vi "Close Notifiers.vi"(8 "error in":errorcluster, 11 "Notifiers":T1) -> (0 "error out":errorcluster)   [LabVIEW 2015, in "Notifiers.lvlib"]
doc: "Releases notifiers"
uses:
  Notifiers.lvlib
  Notifiers.ctl
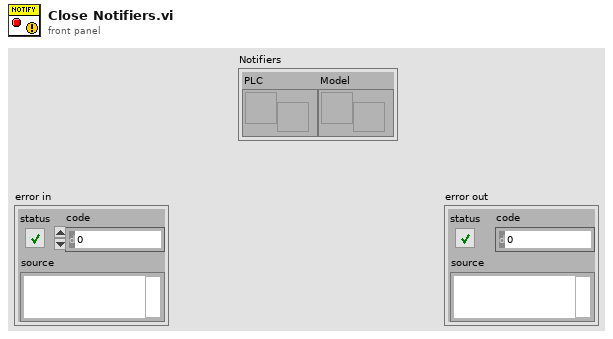
[diagram p1: front panel]
types:
  T1 = typedef "Notifiers.lvlib/Notifiers.ctl" = cluster{"PLC":refnum<notifier>, "Model":refnum<notifier>}
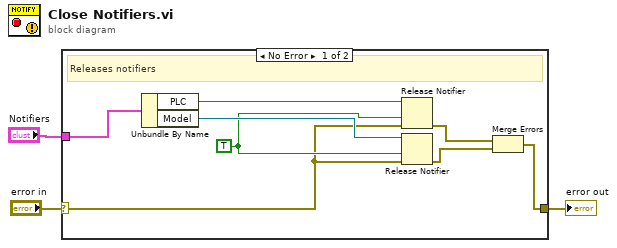
[diagram p0: block diagram]
diagram:
  n1 = case shown="No Error" "error in" {
    selector: "error in" -> [w4 w12]
    tunnel: [w8 w12] -> w2
    tunnel: "Notifiers" -> [w11 _]
    frame No Error {
      w5 = TRUE ("force destroy? (F)")
      # "Releases notifiers"
      n2 = Unbundle By Name(w11) -> ("PLC"=w10:refnum<notifier>, "Model"=w7:refnum<notifier>)
      n3 = Release Notifier(notifier=w10, force destroy? (F)=w5, error in (no error)=w4) -> (error out=w9:errorcluster)  [unwired: 2 out]
      n4 = Release Notifier(notifier=w7, force destroy? (F)=w5, error in (no error)=w4) -> (error out=w6:errorcluster)  [unwired: 2 out]
      n5 = Merge Errors(w9, w6) -> (w8:errorcluster)
    }
    frame Error {
    }
  }
  "error out" <- w2
